vi "MAIN_define_or_reset_ROI.vi"(4 "ROI":T2, 5 "error in":errorcluster, 6 "Reset roi":bool, 7 "Start acquisition":bool, 8 "queue CAMERA":refnum<queue>) -> (0 "error out":errorcluster, 3 "Next task":T1)   [LabVIEW 2015]
uses:
  CONTROLS/Q_camera_element.ctl
  CONTROLS/Q_main_element.ctl
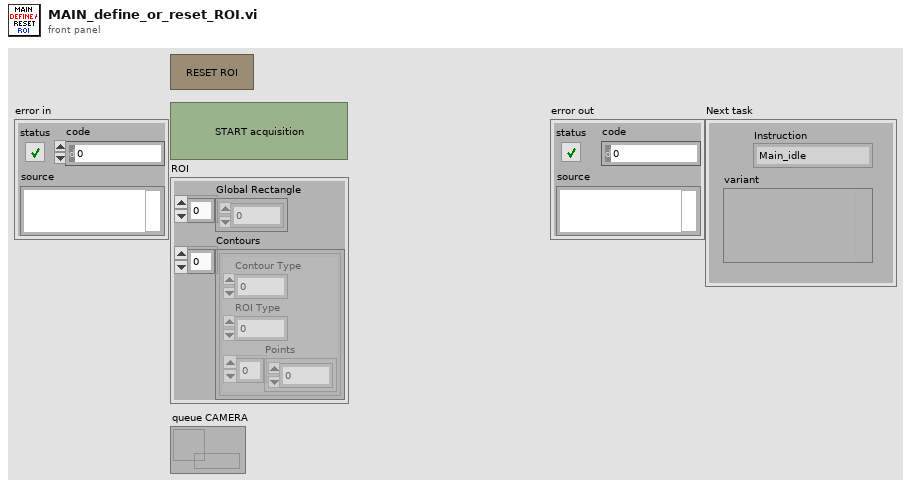
[diagram p1: front panel]
types:
  T1 = typedef "Q_main_element.ctl" = cluster{"variant":variant, "Instruction":enum16{"Main_idle", "Main_initialize", "Main_initialize_TDMS", "Main_initialize_Queue", "Main_error", "Main_DAQ_initialization_results", "Main_ASI_initialization_results", "Main_Piezo_initialization_results", "Main_Valve_initialization_results", "Main_Pump_initialization_results", "Main_CAMERA_initialization_results", "Main_FPGA_initialization_results", "Main_DAQ_error", "Main_ASI_error", "Main_Piezo_error", "Main_CAMERA_error", "Main_Valve_error", "Main_Pump_error", "Main_FPGA_error", "Main_start_acquiring", "Main_not_acquiring", "Main_acquiring", "Main_stop_acquiring", "Main_change_exposure", "Main_change_z_scan_parameters", "Main_define_ROI", "Main_define_mosaic", "Main_read_kinetic_time", "Main_cooler", "Main_read_temperature", "Main_save_XY", "Main_load_XY", "Main_discard_XY", "Main_move_to_XY", "Main_measure_QPD", "Main_autofocus_calibration", "Main_autofocus_initialization", "Main_autofocus_stop", "Main_save_PID", "Main_change_H_valve_position", "Main_two_way_valve", "Main_save_movie", "Main_init_single_scan", "Main_single_scan", "Main_stop_single_scan", "Main_merFISH_illumination_parameters", "Main_merFISH_buffer_probe_list", "Main_merFISH_injections_procedure", "Main_merFISH_save_setpoint", "Main_merFISH_DAPI_parameters", "Main_merFISH_Brightfield_parameters", "Main_merFISH_save_embryo_ROI", "Main_merFISH_init", "Main_merFISH_resume", "Main_merFISH_start_autofocus", "Main_merFISH_open_close_valve_merFISH", "Main_merFISH_open_close_valve_photobleaching", "Main_merFISH_hybridization", "Main_merFISH_move_to_ROI", "Main_merFISH_wait_stabilization", "Main_merFISH_move_to_REF", "Main_merFISH_scan", "Main_merFISH_photobleaching_injection", "Main_merFISH_photobleaching", "Main_merFISH_send_email", "Main_merFISH_close", "Main_STOP"}}
  T2 = cluster{"Global Rectangle":i32[], "Contours":cluster{"Contour Type":u32, "ROI Type":u32, "Points":i32[]}[]}
  T3 = typedef "Q_camera_element.ctl" = cluster{"variant":variant, "Instruction":enum16{"CAMERA_idle", "CAMERA_initialize", "CAMERA_error", "CAMERA_security_stop", "CAMERA_not_acquiring", "CAMERA_acquiring", "CAMERA_start_acquiring", "CAMERA_stop_acquiring", "CAMERA_change_exposure", "CAMERA_define_ROI", "CAMERA_cooler", "CAMERA_acquire_movie", "CAMERA_init_scan", "CAMERA_check_image_scan", "CAMERA_close_scan", "CAMERA_init_merFISH", "CAMERA_start_acquiring_merFISH", "CAMERA_close_scan_merFISH", "CAMERA_close_merFISH", "CAMERA_STOP"}}
  T4 = cluster{"Horizontal Offset":i32, "Vertical Offset":i32, "Horizontal Size":i32, "Vertical Size":i32}
  T5 = cluster{"ROI cluster":cluster{"Horizontal Offset":i32, "Vertical Offset":i32, "Horizontal Size":i32, "Vertical Size":i32}, "Start acquisition":bool}
  T6 = cluster{"Sub Region":cluster{"Horizontal Offset":i32, "Vertical Offset":i32, "Horizontal Size":i32, "Vertical Size":i32}, "Start acquisition":bool}
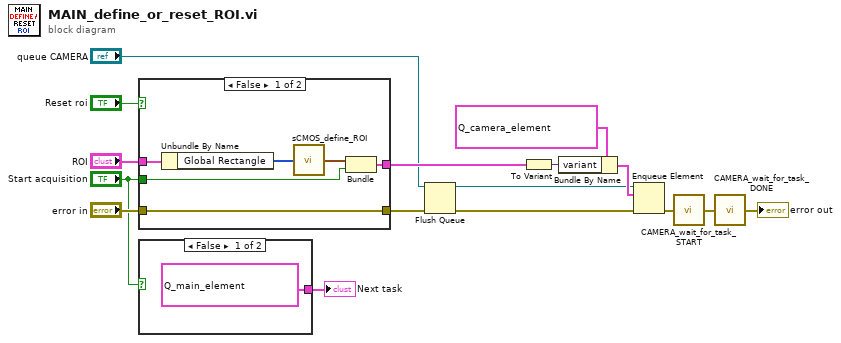
[diagram p0: block diagram]
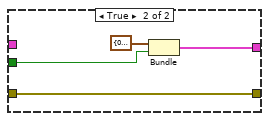
[diagram p2: hidden frame]
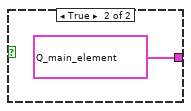
[diagram p3: hidden frame]
diagram:
  n1 = case shown="False" "Reset roi" {
    tunnel: [w22 w24] -> w9
    tunnel: "error in" -> [w17 w26]
    tunnel: [w17 w26] -> w6
    tunnel: "Start acquisition" -> [w21 w25]
    tunnel: "ROI" -> [w18 _]
    frame False {
      n2 = Unbundle By Name(w18) -> ("Global Rectangle"=w20:i32[])
      n3 = call "sCMOS_define_ROI.vi"("Global Rectangle"=w20) -> ("ROI cluster"=w19:T4)
      n4 = Bundle("ROI cluster"=w19, "Start acquisition"=w21) -> (w22:T5)  [unwired: 1 in]
    }
    frame True {
      n5 = Bundle("Sub Region"=T4 {"Horizontal Offset"=0, "Vertical Offset"=0, "Horizontal Size"=2048, "Vertical Size"=2048}, "Start acquisition"=w25) -> (w24:T6)  [unwired: 1 in]
    }
  }
  n6 = case shown="False" "Start acquisition" {
    tunnel: [T1 {"variant"=variant, "Instruction"=enum."Main_not_acquiring"} ("Q_main_element") T1 {"variant"=variant, "Instruction"=enum."Main_acquiring"} ("Q_main_element")] -> w1
    frame False {
    }
    frame True {
    }
  }
  "Next task" <- w1
  n7 = Flush Queue(queue="queue CAMERA", error in (no error)=w6) -> (queue out=w11:refnum<queue>, error out=w4:errorcluster)  [unwired: 1 out]
  n8 = To Variant(anything=w9) -> (Variant=w10:variant)
  n9 = Bundle By Name(cluster=T3 {"variant"=variant, "Instruction"=enum."CAMERA_define_ROI"} ("Q_ANDOR_element"), "variant"=w10) -> (w12:T3)
  n10 = Enqueue Element(queue=w11, element=w12, error in (no error)=w4) -> (error out=w15:errorcluster)  [unwired: 1 in, 2 out]
  n11 = call "CAMERA_wait_for_task_START.vi"("error in"=w15) -> ("error out"=w14:errorcluster)
  n12 = call "CAMERA_wait_for_task_DONE.vi"("error in"=w14) -> ("error out"=→"error out":errorcluster)
